vi "Configure Generation.vi"(8 "error in":errorcluster, 11 "AO DAQmx DC CFG in":refnum<class "AO DAQmx DC CFG.lvclass">) -> (0 "error out":errorcluster, 3 "AO DAQmx DC CFG out":refnum<class "AO DAQmx DC CFG.lvclass">)   [LabVIEW 2024, in "AO DAQmx DC CFG.lvclass"]
uses:
  AO DAQmx DC CFG.lvclass
  DAQmx Base CFG/DAQmx Base CFG.lvclass/DAQmx Base CFG.ctl
  Configurations/CFG Base/CFG Base.lvclass/CFG Base.ctl
  AO DAQmx DC CFG.lvclass/AO DAQmx DC CFG.ctl
  d35ae37b-0a1f-4cf6-9133-ef31fe05ef2e.vi
  <vilib>/DAQmx/write.llb/DAQmx Write (Analog 1D DBL NChan 1Samp).vi
  d35ae37b-0a1f-4cf6-9133-ef31fe05ef2e.vi/a4169a97-72fc-4003-a778-603cf20cafa0.vi
  <vilib>/JDP Science/JSONtext/Find Item.vi
  <vilib>/JDP Science/JSONtext/Next JSON Value.vi
  <vilib>/JDP Science/JSONtext/String Subset.vi
  <vilib>/JDP Science/JSONtext/Parsing/Advance past next JSON Value (inlined COPY).vi
  <vilib>/JDP Science/JSONtext/Parsing/Advance past whitespace.vi
  <vilib>/JDP Science/JSONtext/Parsing/Advance past String.vi
  <vilib>/JDP Science/JSONtext/Parsing/Advance past Number.vi
  <vilib>/JDP Science/JSONtext/Parsing/Advance past Line Ending.vi
  <vilib>/JDP Science/JSONtext/Parsing/Parse Full Path or Item Name.vi
  <vilib>/JDP Science/JSONtext/Parsing/Advance past Array.vi
  <vilib>/JDP Science/JSONtext/Parsing/Advance past Object.vi
  <vilib>/JDP Science/JSONtext/support/Error Cluster From Code.vi
  <vilib>/JDP Science/JSONtext/Offset/Find Item Locations by Path.vi
  <vilib>/JDP Science/JSONtext/JSON text to Variant.vi
  <vilib>/Utility/error.llb/Error Cluster From Error Code.vi
  <vilib>/DAQmx/miscellaneous.llb/DAQmx Fill In Error Info.vi
  <vilib>/JDP Science/JSONtext/LVClass Serializer/JSONtext LVClass Serializer.lvclass
  DAQmx Base CFG/DAQmx Base CFG.lvclass
  <resource>/objmgr/daqmx.rc
  Buffers/BufferWrites1SamDBL/BufferWrites1SamDBL.lvclass
  Configurations/CFG JSON/CFG JSON.lvclass
  Configurations/CFG Base/CFG Base.lvclass
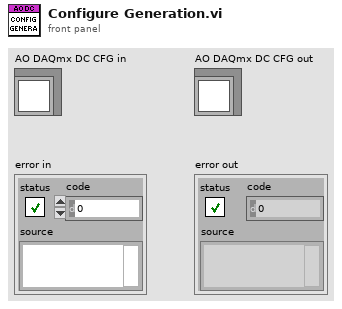
[diagram p1: front panel]
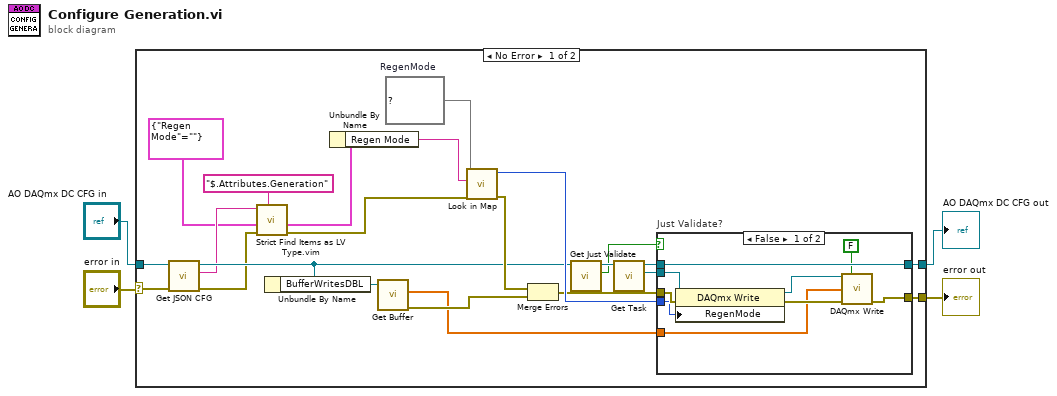
[diagram p0: block diagram]
diagram:
  n1 = case shown="No Error" "error in" {
    selector: "error in" -> [w10 w39]
    tunnel: [w20 w39] -> w2
    tunnel: [w21 w38] -> w3
    tunnel: "AO DAQmx DC CFG in" -> [w25 w38]
    frame No Error {
      w19 = map{string, i32} {"Allow Regeneration"=10097, "Do Not Allow Regeneration"=10158}  # RegenMode
      n2 = call "Get JSON CFG.vi"("CFG JSON in"=w25) -> ("<JSON> CFG"=w8:string, "CFG JSON out"=w15:refnum<class "AO DAQmx DC CFG.lvclass">)  [unwired: 9 in]
      n3 = call "Strict Find Items as LV Type.vim"("$Path or Item Name"="$.Attributes.Generation", "error in"=w10, "Data Type and Default Value"=cluster{"Regen Mode":string} {"Regen Mode"=""}, "<JSON>"=w8) -> ("error out"=w5:errorcluster, "Data out"=w6:cluster{"Regen Mode":string})  [unwired: 5 in, 1 out]
      n4 = Unbundle By Name(w15) -> ("BufferWritesDBL"=w14:refnum<class "BufferWrites1SamDBL.lvclass">)
      n5 = Unbundle By Name(w6) -> ("Regen Mode"=w18:string)
      n6 = call "Get Buffer.vi"("BufferWrites1SamDBL in"=w14) -> ("error out"=w12:errorcluster, "Buffer"=w11:dbl[])  [unwired: 8 in, 1 out]
      n7 = call "Look in Map.vi"("error in"=w5, "Key"=w18, "Map"=w19) -> ("error out"=w17:errorcluster, "Value"=w16:i32)  [unwired: 7 in]
      n8 = Merge Errors(w17, w12) -> (w13:errorcluster)
      n9 = call "Get Just Validate.vi"("CFG Base in"=w15) -> ("Just Validate"=w23:bool, "CFG Base out"=w24:refnum<class "AO DAQmx DC CFG.lvclass">)  [unwired: 9 in]
      n10 = call "Get Task.vi"("DAQmx Base CFG in"=w24) -> ("Task"=w26:refnum<k21>, "DAQmx Base CFG out"=w22:refnum<class "AO DAQmx DC CFG.lvclass">)  [unwired: 9 in]
      n11 = case "Just Validate?" shown="False" w23 {
        tunnel: w13 -> [w35 w36]
        tunnel: w26 -> [w34 _]
        tunnel: w16 -> [w31 _]
        tunnel: w22 -> [w32 w37]
        tunnel: [w32 w37] -> w21
        tunnel: [w30 w36] -> w20
        tunnel: w11 -> [w28 _]
        frame False {
          n12 = property class="DAQmx Write"(reference=w34, error in=w35, "RegenMode"=w31) -> (reference out=w29:refnum<k21>, error out=w33:errorcluster)
          n13 = call-poly <vilib>:"DAQmx Write.vi"("task/channels in"=w29, "auto start"=FALSE, "data"=w28, "error in"=w33) -> ("error out"=w30:errorcluster)  [unwired: 9 in, 2 out]
        }
        frame True {
        }
      }
    }
    frame Error {
    }
  }
  "error out" <- w2
  "AO DAQmx DC CFG out" <- w3
